vi "Laser-Set-Parmeter.vi"(2 "error in (no error)":errorcluster, 3 "LaserHV":u8=20, 5 "LaserFreq":u8=60, 6 "SetLaserEnergy":dbl=0.8, 7 "VISA resource name":refnum<visa-resource-name>) -> (0 "error out":errorcluster, 1 "VISA resource name out":refnum<visa-resource-name>)   [LabVIEW 2013]
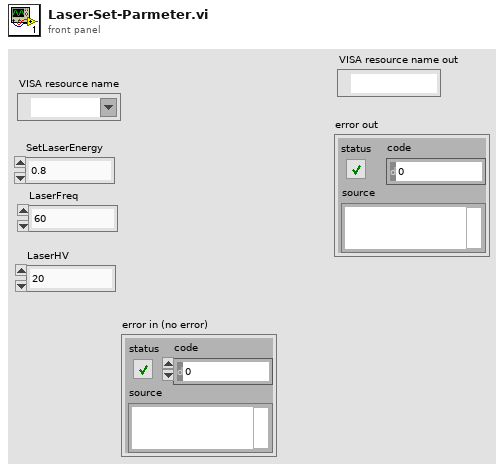
[diagram p1: front panel]
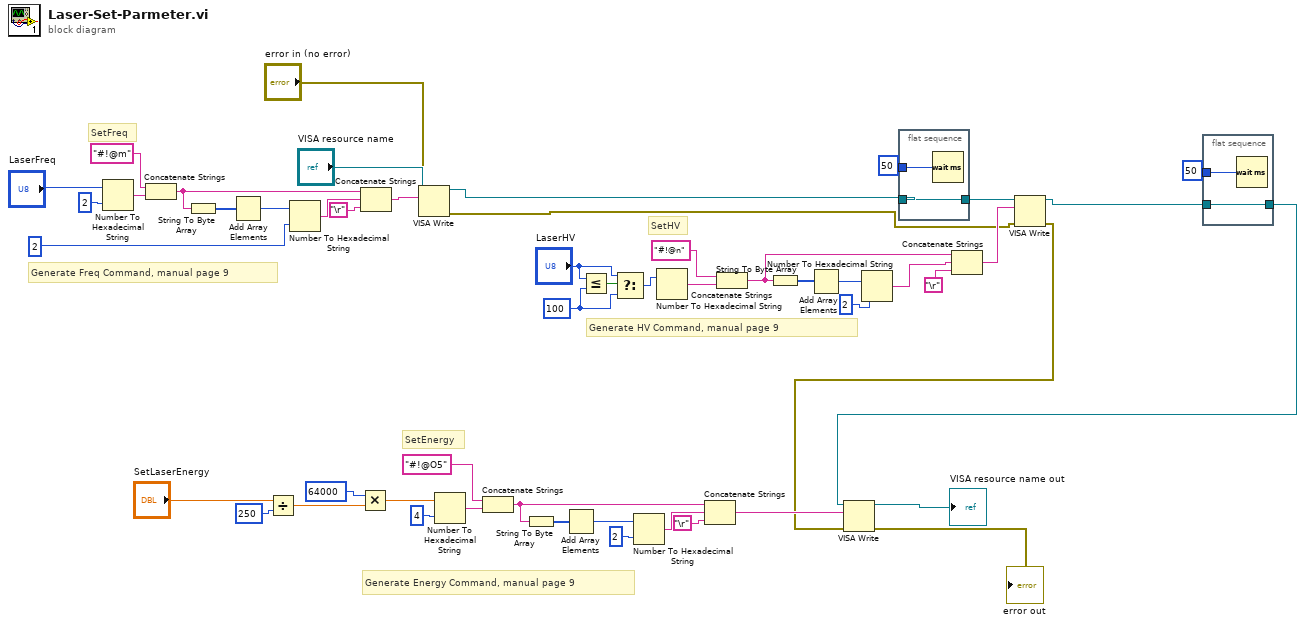
[diagram p0: block diagram]
diagram:
  w38 = u8 100 ("y")
  # "Generate Energy Command, manual page 9"
  # "SetEnergy"
  # "Generate HV Command, manual page 9"
  # "Generate Freq Command, manual page 9"
  # "SetHV"
  # "SetFreq"
  n1 = Number To Hexadecimal String(1:i16 2 ("width (-)"), 2:"LaserFreq") -> (0:w48:string)
  n2 = Concatenate Strings("#!@m" ("string"), w48) -> (w44:string)
  n3 = String To Byte Array(string=w44) -> (unsigned byte array=w47:u8[])
  n4 = Add Array Elements(numeric array=w47) -> (sum=w46:u8)
  n5 = Divide(x="SetLaserEnergy", y=250) -> (x/y=w14:dbl)
  n6 = Number To Hexadecimal String(1:i16 2 ("width (-)"), 2:w46) -> (0:w43:string)
  n7 = Multiply(x=64000, y=w14) -> (x*y=w12:dbl)
  n8 = Concatenate Strings(w44, w43, "\r") -> (w41:string)
  n9 = VISA Write(VISA resource name="VISA resource name", write buffer=w41, error in (no error)="error in (no error)") -> (VISA resource name out=w27:refnum<visa-resource-name>, error out=w3:errorcluster)  [unwired: 1 out]
  n10 = Number To Hexadecimal String(1:i16 4 ("width (-)"), 2:w12) -> (0:w23:string)
  n11 = Concatenate Strings("#!@O5" ("string"), w23) -> (w19:string)
  n12 = String To Byte Array(string=w19) -> (unsigned byte array=w22:u8[])
  n13 = Add Array Elements(numeric array=w22) -> (sum=w21:u8)
  n14 = Less Or Equal?(x="LaserHV", y=w38) -> (x <= y?=w40:bool)
  n15 = Select(t="LaserHV", s=w40, f=w38) -> (s? t:f=w29:u8)
  n16 = Number To Hexadecimal String(1:i16 2 ("width (-)"), 2:w21) -> (0:w18:string)
  n17 = Number To Hexadecimal String(2:w29) -> (0:w36:string)  [unwired: 1 in]
  n18 = Concatenate Strings(w19, w18, "\r") -> (w10:string)
  n19 = Concatenate Strings("#!@n" ("string"), w36) -> (w32:string)
  n20 = String To Byte Array(string=w32) -> (unsigned byte array=w35:u8[])
  n21 = Add Array Elements(numeric array=w35) -> (sum=w34:u8)
  n22 = Number To Hexadecimal String(1:i16 2 ("width (-)"), 2:w34) -> (0:w31:string)
  n23 = flat-sequence {
    tunnel: w27 -> [w52]
    tunnel: [w52] -> w26
    tunnel: u32 50 ("delay before read (ms)") -> [w53]
    frame #0 {
      n24 = Wait (ms)(milliseconds to wait=w53) -> ()  [unwired: 1 out]
    }
  }
  n25 = Concatenate Strings(w32, w31, "\r") -> (w25:string)
  n26 = VISA Write(VISA resource name=w26, write buffer=w25, error in (no error)=w3) -> (VISA resource name out=w8:refnum<visa-resource-name>, error out=w2:errorcluster)  [unwired: 1 out]
  n27 = VISA Write(VISA resource name=w7, write buffer=w10, error in (no error)=w2) -> (VISA resource name out=→"VISA resource name out":refnum<visa-resource-name>, error out=→"error out":errorcluster)  [unwired: 1 out]
  n28 = flat-sequence {
    tunnel: w8 -> [w54]
    tunnel: [w54] -> w7
    tunnel: u32 50 ("delay before read (ms)") -> [w55]
    frame #0 {
      n29 = Wait (ms)(milliseconds to wait=w55) -> ()  [unwired: 1 out]
    }
  }
